vi "Get Pixel Coordinates in ROI.vi"(5 "Max Y (default: any)":i32=2147483647, 7 "Max X (default: any)":i32=2147483647, 8 "Error In":errorcluster, 11 "ROI":T1 {"Contours"."Type" items=["No Selection", "Point", "Line", "Rectangle", "Oval", "Polygon", "Freehand Region", "Annulus", "Unused2", "Unused3", "Broken Line", "Freehand Line", "Rotated Rectangle"]}) -> (0 "Error Out":errorcluster, 3 "Pixels in ROI":cluster{"X":i32, "Y":i32}[](array[cluster]))   [LabVIEW 2021, in "Image.lvlib"]
uses:
  Image.lvlib
  <vilib>/vision/NI_Vision_Development_Module.lvlib
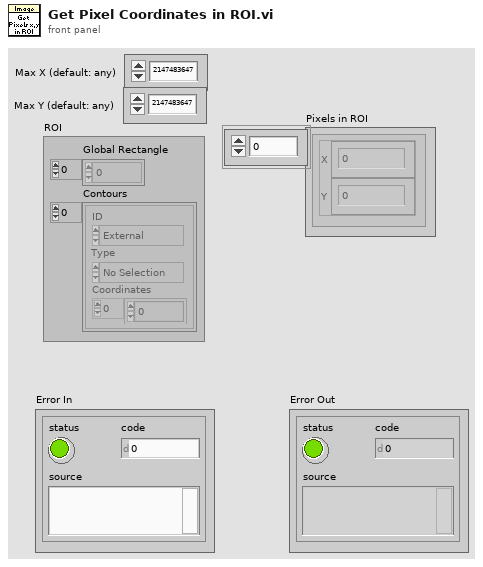
[diagram p1: front panel]
types:
  T1 = typedef "ROI Descriptor" = cluster{"Global Rectangle":i32[], "Contours":cluster{"ID":enum32{"External", "Internal"}, "Type":u32, "Coordinates":i32[]}[]}
  T2 = typedef "Image Type" = u32
  T3 = typedef "IMAQ Image.ctl" = refnum<image>
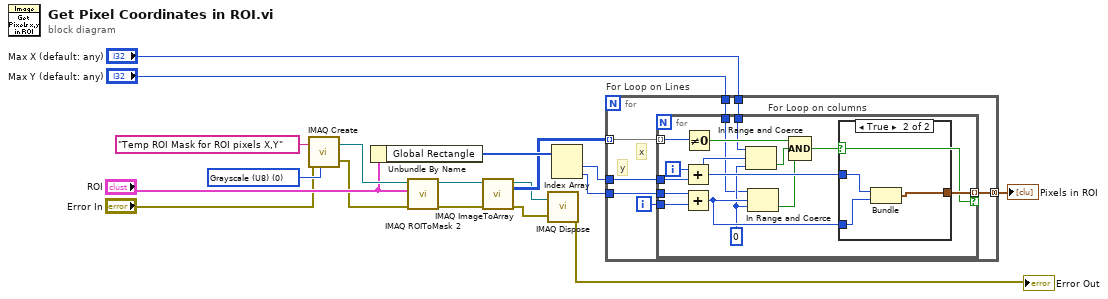
[diagram p0: block diagram]
diagram:
  w16 = T2 0 items=["Grayscale (U8)", "Grayscale (I16)", "Grayscale (SGL)", "Complex (CSG)", "RGB (U32)", "HSL (U32)", "RGB (U64)", "Grayscale (U16)"] ("Image Type")
  n1 = call "IMAQ Create"("Image Name"="Temp ROI Mask for ROI pixels X,Y", "Image Type"=w16, "error in (no error)"="Error In") -> ("New Image"=w17:T3, "error out"=w4:errorcluster)  [unwired: 2 in]
  n2 = Unbundle By Name("ROI") -> ("Global Rectangle"=w13:i32[])
  n3 = call "IMAQ ROIToMask 2"("error in (no error)"=w4, "ROI Descriptor"="ROI", "Image"=w17) -> ("error out"=w14:errorcluster, "Image Out"=w8:T3)  [unwired: 6 in, 1 out]
  n4 = call "IMAQ ImageToArray"("error in (no error)"=w14, "Image"=w8) -> ("error out"=w9:errorcluster, "Image Pixels (U8)"=w12:u8[][])  [unwired: 2 in, 3 out]
  n5 = call "IMAQ Dispose"("Image"=w8, "error in (no error)"=w9) -> ("error out"=→"Error Out":errorcluster)  [unwired: 4 in]
  n6 = Index Array(array=w13) -> (element #1=w11:i32, element #2=w10:i32)  [unwired: 2 in]
  n7 = for "For Loop on Lines" {
    tunnel: w12 -> [w24] mode=indexing
    tunnel: w10 -> [w23]
    tunnel: w11 -> [w22]
    tunnel: [w21] -> w2 mode=concatenating
    tunnel: "Max X (default: any)" -> [w19]
    tunnel: "Max Y (default: any)" -> [w18]
    i -> [w20]
    # "x"
    # "y"
    n8 = for "For Loop on columns" {
      tunnel: w24 -> [w39] mode=indexing
      tunnel: w23 -> [w33]
      tunnel: w22 -> [w35]
      tunnel: [w38] -> w21 mode=indexing if=w27
      tunnel: w20 -> [w34]
      tunnel: w19 -> [w26]
      tunnel: w18 -> [w25]
      i -> [w36]
      w29 = 0 ("lower limit")
      n9 = Add(x=w36, y=w35) -> (x+y=w32:i32)
      n10 = Add(x=w33, y=w34) -> (x+y=w30:i32)
      n11 = Not Equal To 0?(x=w39) -> (x != 0?=w37:bool)
      n12 = In Range and Coerce(upper limit=w26, x=w32, lower limit=w29) -> (In Range?=w31:bool)  [unwired: 1 out]
      n13 = In Range and Coerce(upper limit=w25, x=w30, lower limit=w29) -> (In Range?=w28:bool)  [unwired: 1 out]
      n14 = Compound Arithmetic op=AND(w37, w31, w28) -> (w27:bool)
      n15 = case shown="True" w27 {
        tunnel: w32 -> [_ w42]
        tunnel: w30 -> [_ w41]
        tunnel: [_ w40] -> w38
        frame False {
        }
        frame True {
          n16 = Bundle(w42, w41) -> (w40:cluster{i32, i32})  [unwired: 1 in]
        }
      }
    }
  }
  "Pixels in ROI" <- w2
